vi "mules_exit_exe.vi"(1 "error in (no error)":errorcluster, 2 "Quit? (T)":bool=TRUE) -> ()   [LabVIEW 2013]
doc: "Exits the environment only if the VI is run in the RTE.\nIf an error is wired in, displays a message before exiting."
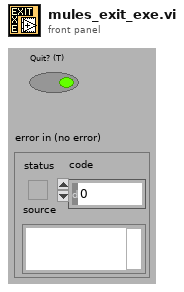
[diagram p1: front panel]
types:
  T1 = enum32{"invalid app kind", "Development System", "Run Time System", "Student Edition", "Embedded LabVIEW", "Evaluation", "Custom"}
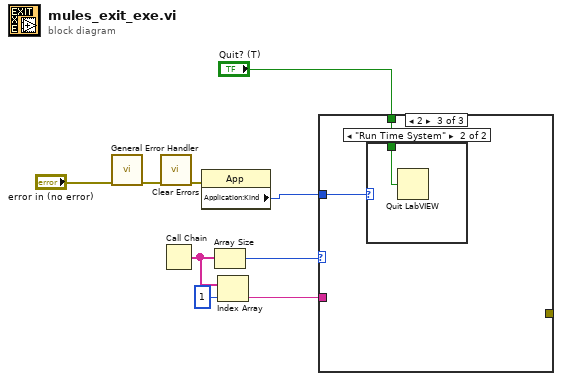
[diagram p0: block diagram]
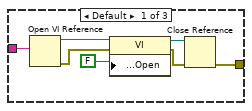
[diagram p2: hidden frame]
diagram:
  n1 = call <vilib>:"General Error Handler.vi"("error in (no error)"="error in (no error)") -> ("error out"=w6:errorcluster)  [unwired: 1 in, 13 out]
  n2 = call <vilib>:"Clear Errors.vi"("error in (no error)"=w6) -> ("error out"=w5:errorcluster)  [unwired: 6 out]
  n3 = Call Chain() -> (call chain=w3:string[])
  n4 = property class="App"(error in=w5) -> ("Application:Kind"=w9:T1)  [unwired: 1 in, 2 out]
  n5 = Array Size(array=w3) -> (size(s)=w4:i32)
  n6 = Index Array(array=w3, index=1) -> (element=w1:string)
  n7 = case shown="2" w4 {
    tunnel: w9 -> [_ _ w18]
    tunnel: "Quit? (T)" -> [_ _ w17]
    tunnel: [w13 _ _] -> _
    tunnel: w1 -> [w12 _ _]
    frame Default {
      n8 = Open VI Reference(vi path=w12) -> (vi reference=w11:refnum<vi>, error out=w10:errorcluster)  [unwired: 1 in, 4 out]
      n9 = property class="VI"(reference=w11, error in=w10, "Front Panel Window:Open"=FALSE) -> (reference out=w15:refnum<vi>, error out=w14:errorcluster)
      n10 = Close Reference(reference=w15, error in (no error)=w14) -> (error out=w13:errorcluster)
    }
    frame 1 {
    }
    frame 2 {
      n11 = case shown="\"Run Time System\"" w18 {
        tunnel: w17 -> [_ w19]
        frame Default {
        }
        frame "Run Time System" {
          n12 = Quit LabVIEW(quit? (T)=w19) -> ()
        }
      }
    }
  }
